vi "MP_LaunchMatlabScript4 (1).vi"(6 "Remove ML msg (T)":bool=TRUE, 8 "error in (no error)":errorcluster, 11 "matlab script path":path) -> (0 "error out":errorcluster, 2 "standard error":string, 3 "standard output":string, 4 "OS Name":string, 5 "computed command line":string, 7 "Apple Silicon":bool)   [LabVIEW 2025]
doc: "Launch matlab with the script passed as parameter. \nThe script and the VI MUST be in the same directory!\n\nWorks on OSX, Windows and Linux\n\nOn OSX, search for the latest release of matlab, see diagram.\nOn Windows, assume \"matlab\" command exists.\nOn Linux, assume Ubuntu (salles CO) and current 2013 \"matlab\" CMD - not stested recently....\n\nThere is demo script if needed, see the diagram to activate it.\n\nadded stderr and stdout error parsing to remove \"warnings\", adapt as necessary.\n\nChS. 2013-25, updated to use '-batch' instead of '-r'"
uses:
  <vilib>/Utility/sysdir.llb/System Directory Type.ctl
panel:
  in  "To be removed from ML stdout":string[](array[string])=["[\bWarning: Command line argument -sd has already been specified.\n-useStartupFolderPref will be ignored.]\b "]
  out "ML Apple Silicon":bool
  out "ML intel":bool
  out "Contents/MacOS":bool
  in  "To be removed from ML stderr":string[](array[string])=["CoreText note:", "Class WebSwapCGLLayer is implemented in both", "CodeCache is full", "Try increasing the code cache size using -XX:"]
  out "is shortcut":bool
  out "is directory":bool
  # "Since ML 2018 use \"-batch\""
  # "Added script path"
  # "Added ML 2023 Intel/AS suppport + msg parsing"
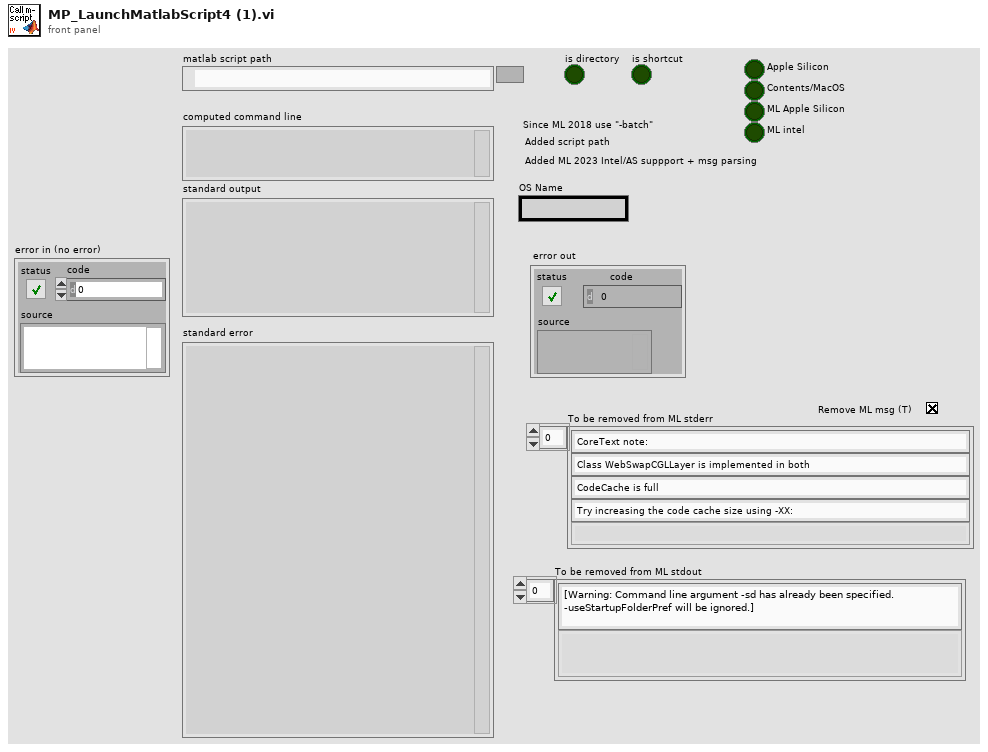
[diagram p1: front panel]
types:
  T1 = enum16{"open", "replace", "create", "open or create", "replace or create", "replace or create with confirmation"}
  T2 = typedef "System Directory Type.ctl" = i32
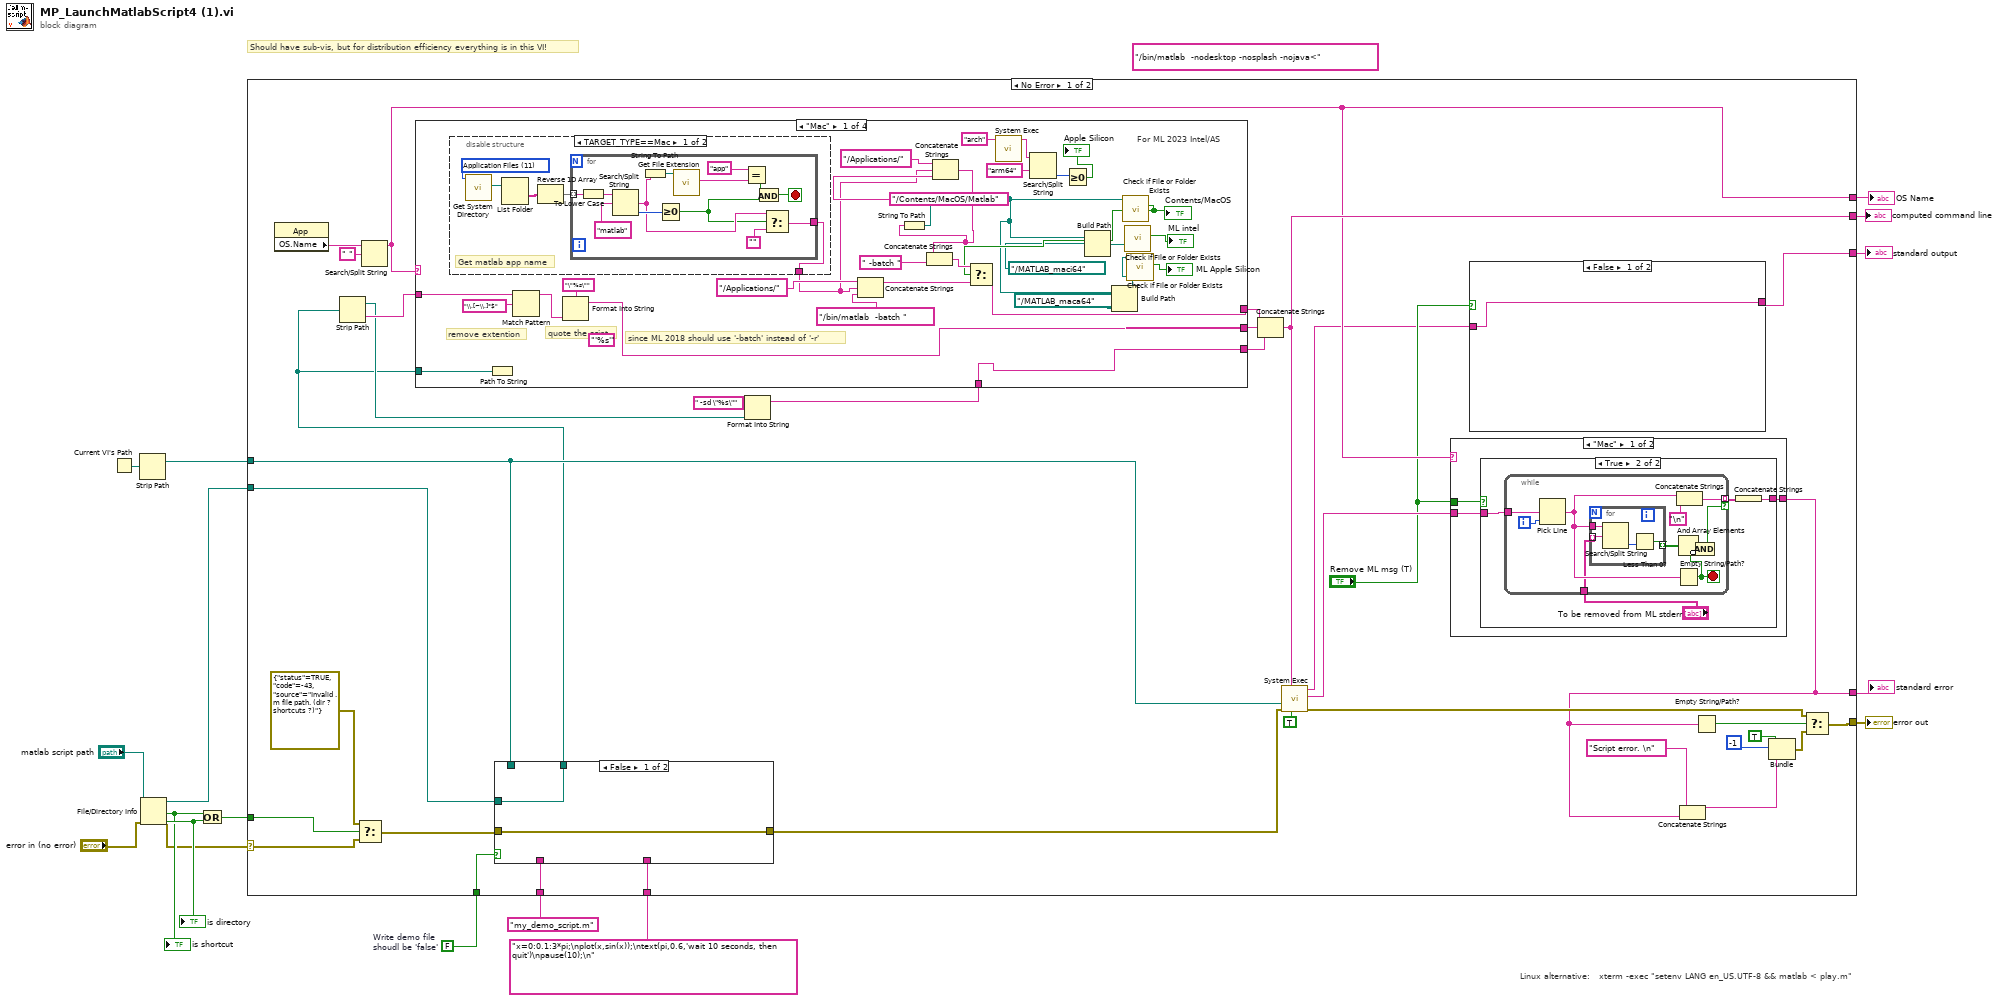
[diagram p0: block diagram]
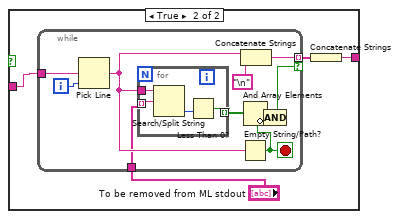
[diagram p2: hidden frame]
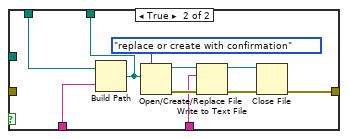
[diagram p5: hidden frame]
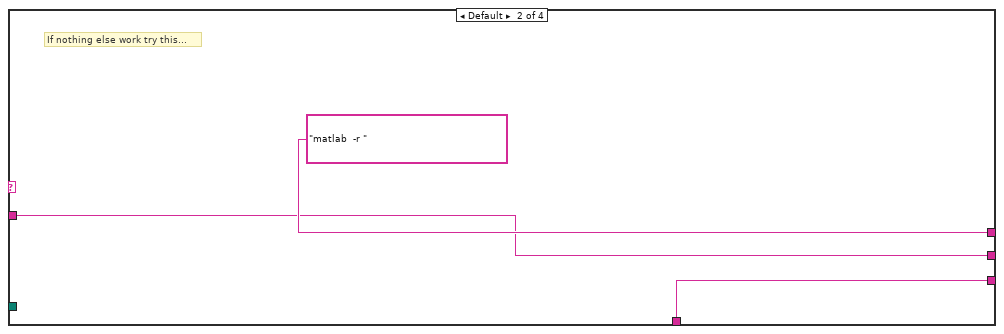
[diagram p7: hidden frame]
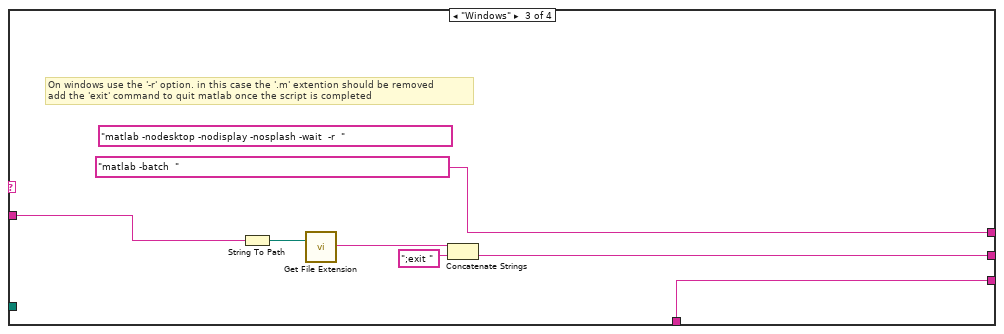
[diagram p8: hidden frame]
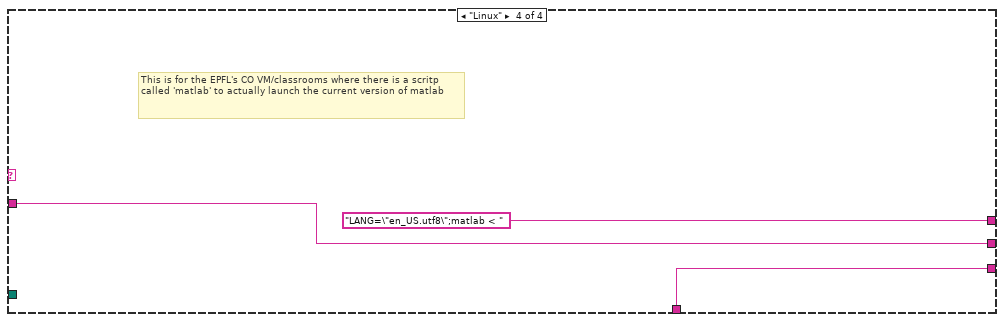
[diagram p9: hidden frame]
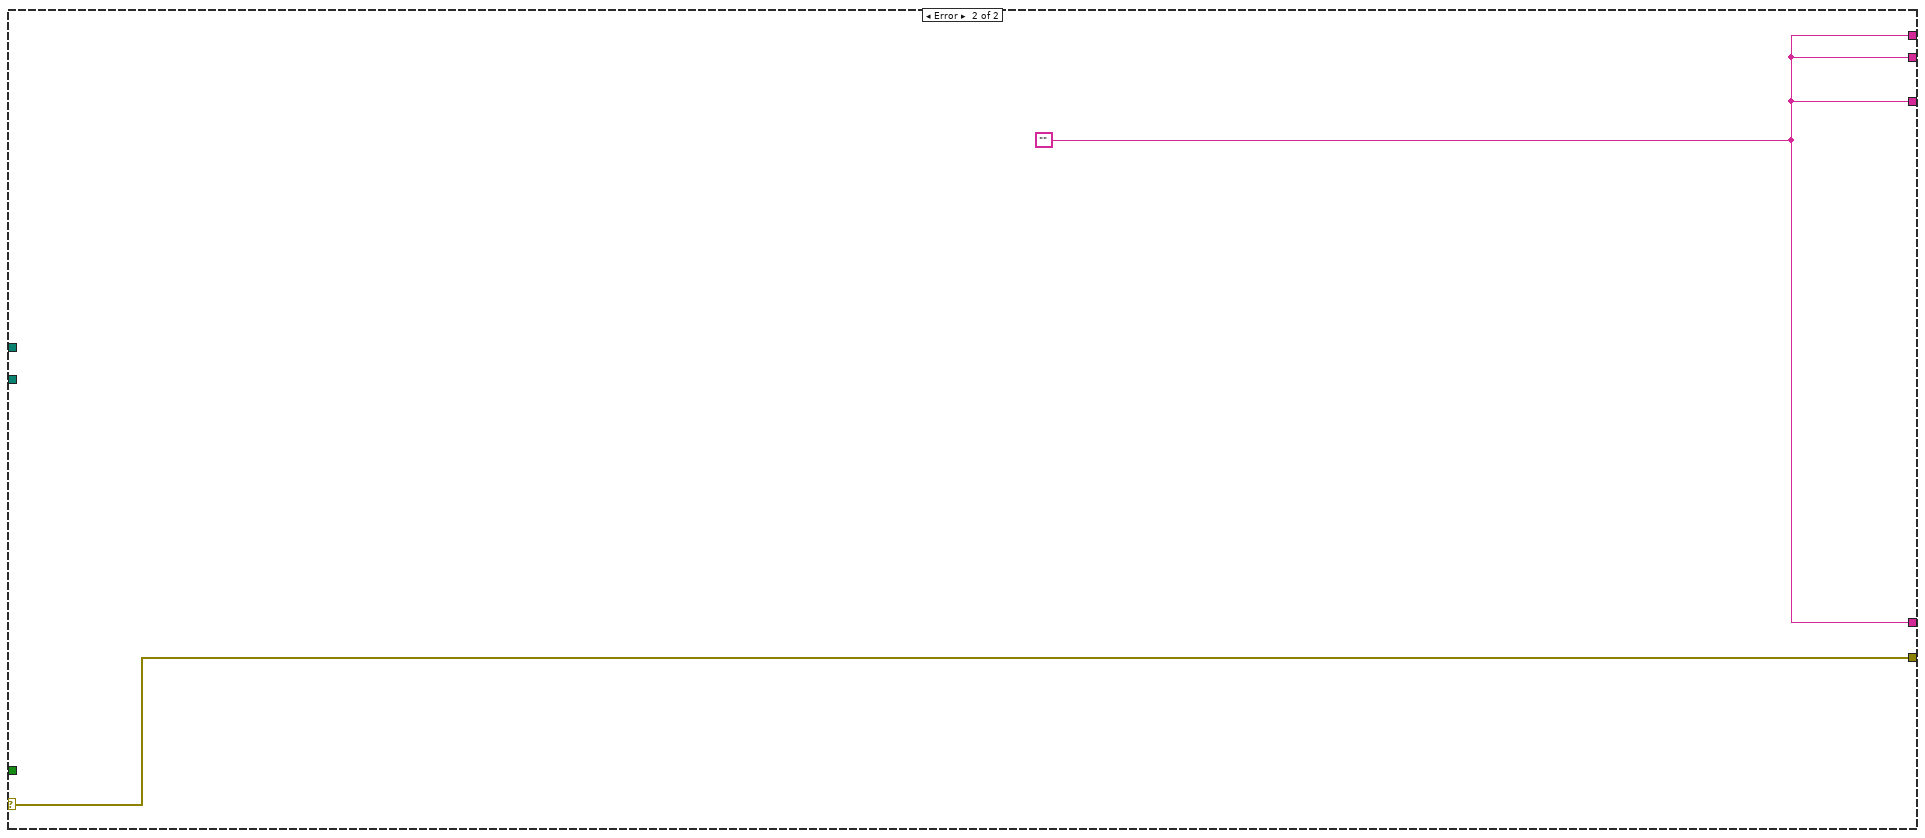
[diagram p10: hidden frame]
diagram:
  (unwired) "/bin/matlab  -nodesktop -nosplash -nojava<" ("name or relative path")
  w10 = FALSE  # Write demo file shoudl be 'false'
  # "Should have sub-vis, but for distribution efficiency everything is in this VI!"
  # "Linux alternative:   xterm -exec \"setenv LANG en_US.UTF-8 && matlab < play.m\""
  n1 = Current VI's Path() -> (path=w9:path)
  n2 = Strip Path(path=w9) -> (stripped path=w8:path)  [unwired: 1 out]
  n3 = File/Directory Info(path="matlab script path", error in="error in (no error)") -> (path out=w6:path, directory=w5:bool, error out=w1:errorcluster, shortcut=w4:bool)  [unwired: 3 out]
  "is directory" <- w5
  "is shortcut" <- w4
  n4 = Or(x=w4, y=w5) -> (x .or. y?=w3:bool)
  n5 = case shown="No Error" w1 {
    selector: w1 -> [w53 w170]
    tunnel: [w18 w169] -> w17
    tunnel: [w24 w169] -> w16
    tunnel: [w46 w170] -> w15
    tunnel: [w49 w169] -> w14
    tunnel: [w26 w169] -> w13
    tunnel: "x=0:0.1:3*pi;\nplot(x,sin(x));\ntext(pi,0.6,'wait 10 seconds, then quit')\npause(10);\n" ("text") -> [w37 _]
    tunnel: "my_demo_script.m" ("name or relative path") -> [w36 _]
    tunnel: w10 -> [w35 _]
    tunnel: w8 -> [w33 _]
    tunnel: w6 -> [w27 _]
    tunnel: w3 -> [w29 _]
    frame No Error {
      n6 = property class="App"() -> ("OS.Name"=w39:string)  [unwired: 2 in, 2 out]
      n7 = Select(t=errorcluster {"status"=TRUE, "code"=-43, "source"="Invalid .m file path. (dir ? shortcuts ?)"} ("error constant"), s=w29, f=w53) -> (s? t:f=w51:errorcluster)
      n8 = Search/Split String(string=w39, search string/char (-)=" ") -> (substring before match=w26:string)  [unwired: 1 in, 2 out]
      n9 = case shown="False" w35 {
        tunnel: [w97 w103] -> w28
        tunnel: w33 -> [_ w101]
        tunnel: w51 -> [w97 _]
        tunnel: w37 -> [_ w100]
        tunnel: w36 -> [_ w99]
        tunnel: [w96 w98] -> w21
        tunnel: w27 -> [w96 _]
        frame False {
        }
        frame True {
          n10 = Build Path(base path=w101, name or relative path=w99) -> (appended path=w98:path)
          n11 = Open/Create/Replace File(file path (use dialog)=w98, operation (0:open)=T1."replace or create with confirmation") -> (refnum out=w104:refnum<file>, error out=w107:errorcluster)  [unwired: 4 in, 1 out]
          n12 = Write to Text File(file (use dialog)=w104, text=w100, error in=w107) -> (refnum out=w105:refnum<file>, error out=w106:errorcluster)  [unwired: 1 in, 1 out]
          n13 = Close File(refnum=w105, error in=w106) -> (error out=w103:errorcluster)  [unwired: 1 out]
        }
      }
      n14 = Strip Path(path=w21) -> (stripped path=w31:path, name=w32:string)
      n15 = Format Into String(format string=" -sd \"%s\"", w31) -> (resulting string=w23:string)  [unwired: 2 in, 1 out]
      n16 = case shown="\"Mac\"" w26 {
        tunnel: [w129 "matlab  -r " ("name or relative path") "matlab -batch  " ("name or relative path") "LANG=\"en_US.utf8\";matlab < "] -> w50
        tunnel: w32 -> [w136 w157 w164 w167]
        tunnel: [w109 w157 w161 w167] -> w40
        tunnel: w23 -> [w108 w156 w159 w166]
        tunnel: [w108 w156 w159 w166] -> w22
        tunnel: w21 -> [w111 _ _ _]
        frame "Mac" {
          (unwired) "'%s'" ("format string")
          # "For ML 2023 Intel/AS"
          # "since ML 2018 should use '-batch' instead of '-r'"
          # "quote the scipt"
          # "remove extention"
          n17 = disable-structure shown="TARGET_TYPE==Mac" {
            disable-tunnel: [w138 _] -> w131
            frame condition #0 (active) {
              w142 = T2 11 items=["User Home"=0, "User Desktop"=1, "User Documents"=2, "User Application Data"=3, "User Preferences"=4, "User Temporary"=5, "Public Documents"=6, "Public Application Data"=7, "Public Preferences"=8, "Public Cache"=13, "System Core Libraries"=9, "System Installed Libraries"=10, "Application Files"=11, "Boot Volume Root"=12] ("system directory type")
              # "Get matlab app name"
              n18 = call <vilib>:"Get System Directory.vi"("system directory type"=w142) -> ("system directory"=w139:path)  [unwired: 10 in]
              n19 = List Folder(path=w139) -> (folder names=w141:string[])  [unwired: 3 in, 3 out]
              n20 = Reverse 1D Array(array=w141) -> (reversed array=w140:string[])
              n21 = for {
                tunnel: w140 -> [w155] mode=indexing
                tunnel: [w146] -> w138
                stop <- w148 stop-if-true
                n22 = To Lower Case(string=w155) -> (all lower case string=w154:string)
                n23 = Search/Split String(string=w154, search string/char (-)="matlab") -> (match + rest of string=w145:string, offset of match=w152:i32)  [unwired: 1 in, 1 out]
                n24 = String To Path(string=w145) -> (path=w151:path)
                n25 = Greater Or Equal To 0?(x=w152) -> (x >= 0?=w144:bool)
                n26 = call <vilib>:"Get File Extension.vi"("file"=w151) -> ("lowercase file extension"=w149:string)  [unwired: 6 in, 4 out]
                n27 = Equal?(x="app", y=w149) -> (x = y?=w147:bool)
                n28 = And(x=w147, y=w144) -> (x .and. y?=w148:bool)
                n29 = Select(t=w145, s=w144, f="") -> (s? t:f=w146:string)
              }
            }
            frame condition #1 {
            }
          }
          n30 = Path To String(path=w111) -> ()  [unwired: 1 out]
          n31 = Match Pattern(string=w136, regular expression="\\.[~\\.]*$") -> (before substring=w135:string)  [unwired: 1 in, 3 out]
          n32 = Format Into String(format string="\"%s\"", w135) -> (resulting string=w109:string)  [unwired: 2 in, 1 out]
          n33 = Concatenate Strings("/Applications/" ("name or relative path"), w131, "/bin/matlab  -batch " ("name or relative path")) -> (w130:string)
          n34 = Concatenate Strings("/Applications/" ("name or relative path"), w131, "/Contents/MacOS/Matlab" ("string")) -> (w126:string)
          n35 = String To Path(string=w126) -> (path=w112:path)
          n36 = Concatenate Strings(w126, " -batch " ("string")) -> (w125:string)
          n37 = call <vilib>:"System Exec.vi"("command line"="arch") -> ("standard output"=w123:string)  [unwired: 7 in, 3 out]
          n38 = Search/Split String(string=w123, search string/char (-)="arm64") -> (offset of match=w121:i32)  [unwired: 1 in, 2 out]
          n39 = Greater Or Equal To 0?(x=w121) -> (x >= 0?=→"Apple Silicon":bool)
          n40 = Build Path(base path=w112, name or relative path=path "../MATLAB_maci64") -> (appended path=w118:path)
          n41 = Build Path(base path=w112, name or relative path=path "../MATLAB_maca64") -> (appended path=w115:path)
          n42 = call <vilib>:"Check if File or Folder Exists.vi"("path"=w112) -> ("file or folder exists?"=w119:bool)  [unwired: 8 in, 2 out]
          "Contents/MacOS" <- w119
          n43 = Select(t=w125, s=w119, f=w130) -> (s? t:f=w129:string)
          n44 = call <vilib>:"Check if File or Folder Exists.vi"("path"=w118) -> ("file or folder exists?"=→"ML intel":bool)  [unwired: 8 in, 2 out]
          n45 = call <vilib>:"Check if File or Folder Exists.vi"("path"=w115) -> ("file or folder exists?"=→"ML Apple Silicon":bool)  [unwired: 8 in, 2 out]
        }
        frame Default {
          # "If nothing else work try this..."
        }
        frame "Windows" {
          (unwired) "matlab -nodesktop -nodisplay -nosplash -wait  -r  " ("name or relative path")
          # "On windows use the '-r' option. in this case the '.m' extention should be removed\nadd the 'exit' command to quit matlab once the script is completed"
          n46 = String To Path(string=w164) -> (path=w163:path)
          n47 = call <vilib>:"Get File Extension.vi"("file"=w163) -> ("filename without extension"=w162:string)  [unwired: 6 in, 4 out]
          n48 = Concatenate Strings(w162, ";exit " ("string")) -> (w161:string)
        }
        frame "Linux" {
          # "This is for the EPFL's CO VM/classrooms where there is a scritp called 'matlab' to actually launch the current version of matlab"
        }
      }
      n49 = Concatenate Strings(w50, w40, w22) -> (w49:string)
      n50 = call <vilib>:"System Exec.vi"("run minimized? (F)"=TRUE, "error in (no error)"=w28, "working directory"=w33, "command line"=w49) -> ("error out"=w47:errorcluster, "standard error"=w25:string, "standard output"=w19:string)  [unwired: 4 in, 1 out]
      n51 = case shown="\"Mac\"" w26 {
        tunnel: "Remove ML msg (T)" -> [w75 _]
        tunnel: w25 -> [w74 w95]
        tunnel: [w73 w95] -> w24
        frame "Mac" {
          n52 = case shown="True" w75 {
            tunnel: w74 -> [w76 w78]
            tunnel: [w76 w77] -> w73
            frame False {
            }
            frame True {
              n53 = while {
                tunnel: w78 -> [w89]
                tunnel: [w84] -> w80 mode=indexing if=w82
                tunnel: "To be removed from ML stderr" -> [w87]
                i -> [w90]
                stop <- w81 stop-if-true
                n54 = Pick Line(multi-line string=w89, line index=w90) -> (output string=w88:string)  [unwired: 1 in]
                n55 = for {
                  tunnel: [w93] -> w86 mode=indexing
                  tunnel: w88 -> [w92]
                  tunnel: w87 -> [w91] mode=indexing
                  n56 = Search/Split String(string=w92, search string/char (-)=w91) -> (offset of match=w94:i32)  [unwired: 1 in, 2 out]
                  n57 = Less Than 0?(x=w94) -> (x < 0?=w93:bool)
                }
                n58 = And Array Elements(Boolean array=w86) -> (logical AND=w85:bool)
                n59 = Empty String/Path?(string/path=w88) -> (empty?=w81:bool)
                n60 = Concatenate Strings(w88, "\n") -> (w84:string)
                n61 = Compound Arithmetic op=AND(w85, invert w81) -> (w82:bool)
              }
              n62 = Concatenate Strings(w80) -> (w77:string)
            }
          }
        }
        frame Default {
        }
      }
      n63 = case shown="False" "Remove ML msg (T)" {
        tunnel: [w54 w56] -> w18
        tunnel: w19 -> [w54 w55]
        frame False {
        }
        frame True {
          n64 = while {
            tunnel: w55 -> [w67]
            tunnel: [w62] -> w58 mode=indexing if=w60
            tunnel: "To be removed from ML stdout" -> [w65]
            i -> [w68]
            stop <- w59 stop-if-true
            n65 = Pick Line(multi-line string=w67, line index=w68) -> (output string=w66:string)  [unwired: 1 in]
            n66 = for {
              tunnel: [w71] -> w64 mode=indexing
              tunnel: w66 -> [w70]
              tunnel: w65 -> [w69] mode=indexing
              n67 = Search/Split String(string=w70, search string/char (-)=w69) -> (offset of match=w72:i32)  [unwired: 1 in, 2 out]
              n68 = Less Than 0?(x=w72) -> (x < 0?=w71:bool)
            }
            n69 = And Array Elements(Boolean array=w64) -> (logical AND=w63:bool)
            n70 = Empty String/Path?(string/path=w66) -> (empty?=w59:bool)
            n71 = Concatenate Strings(w66, "\n") -> (w62:string)
            n72 = Compound Arithmetic op=AND(w63, invert w59) -> (w60:bool)
          }
          n73 = Concatenate Strings(w58) -> (w56:string)
        }
      }
      n74 = Concatenate Strings("Script error. \n" ("source"), w24) -> (w42:string)
      n75 = Empty String/Path?(string/path=w24) -> (empty?=w48:bool)
      n76 = Bundle("status"=TRUE, "code"=-1, w42) -> (w45:cluster{"status":bool, "code":i32, string})  [unwired: 1 in]
      n77 = Select(t=w47, s=w48, f=w45) -> (s? t:f=w46:errorcluster)
    }
    frame Error {
      w169 = "" ("standard error")
    }
  }
  "standard output" <- w17
  "standard error" <- w16
  "error out" <- w15
  "computed command line" <- w14
  "OS Name" <- w13
